vi "Add Parameter Channels with Definitions.vi"(6 "direction":T4, 8 "error in":errorcluster, 10 "parameters":T3(array[cluster]), 11 "message in":T1 format="%.0x") -> (0 "error out":errorcluster, 3 "message out":T1 format="%.0x")   [LabVIEW 2020, in "Ballard MIL-STD-1553 Scripting.lvlib"]
uses:
  Ballard MIL-STD-1553 Scripting.lvlib
  Shared/Direction.ctl
  <vilib>/NI VeriStand/Custom Device API/Custom Device Item Ref.ctl
  Shared/Parameter Definition.ctl
  <vilib>/NI VeriStand/Custom Device API/Custom Device Channel Type.ctl
  <vilib>/NI VeriStand/Custom Device API/Custom Device Channel.ctl
  <vilib>/NI VeriStand/Custom Device API/Custom Device API.lvlib
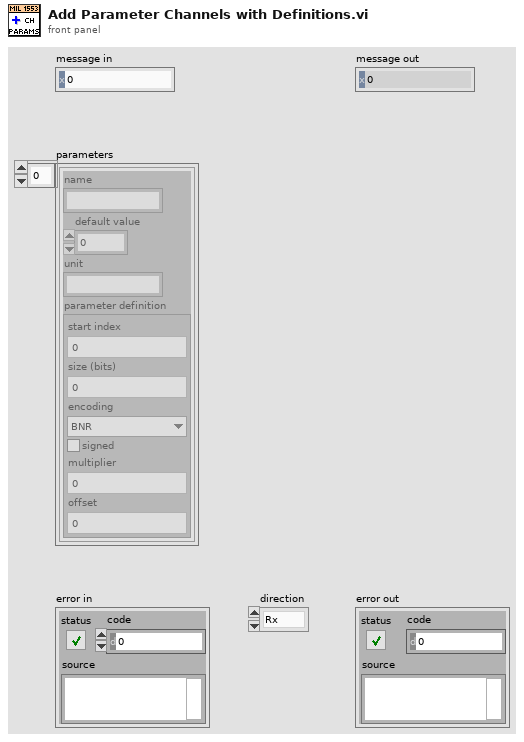
[diagram p1: front panel]
types:
  T1 = typedef "Custom Device API.lvlib/Custom Device Item Ref.ctl" = u64
  T2 = typedef "Parameter Definition.ctl" = cluster{"start index":i32, "size (bits)":i32, "encoding":enum16{"BNR", "BCD", "Discrete"}, "signed":bool, "multiplier":dbl, "offset":dbl}
  T3 = cluster{"name":string, "default value":dbl, "unit":string, "parameter definition":T2}[]
  T4 = typedef "Direction.ctl" = enum16{"Rx", "Tx"}
  T5 = typedef "Custom Device API.lvlib/Custom Device Channel Type.ctl" = enum16{"Input", "Output"}
  T6 = typedef "Custom Device API.lvlib/Custom Device Channel.ctl" = cluster{"Type":T5, "Units":string, "Default Value":dbl, "Faultable":bool, "Scalable":bool}
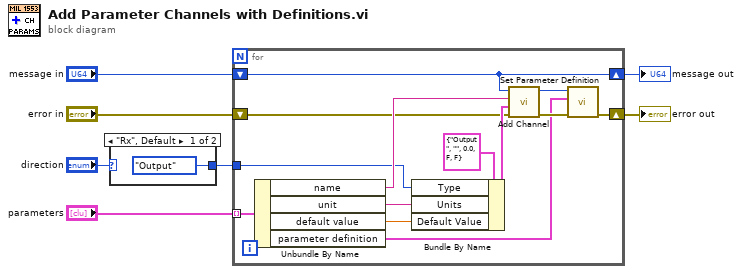
[diagram p0: block diagram]
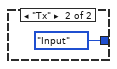
[diagram p2: hidden frame]
diagram:
  n1 = case shown="\"Rx\", Default" "direction" {
    tunnel: [Custom_Device_Channel_Type."Output" ("Type") Custom_Device_Channel_Type."Input" ("Type")] -> w1
    frame "Rx", Default {
    }
    frame "Tx" {
    }
  }
  n2 = for {
    shift-right: [w13] -> w7
    shift-left: "message in" -> [w13]
    tunnel: "parameters" -> [w22] mode=indexing
    shift-right: [w11] -> w6
    shift-left: "error in" -> [w12]
    tunnel: w1 -> [w10]
    n3 = Unbundle By Name(w22) -> ("name"=w18:string, "unit"=w20:string, "default value"=w19:dbl, "parameter definition"=w14:T2)
    n4 = Bundle By Name(cluster=T6 {"Type"=enum."Output", "Units"="", "Default Value"=0.0, "Faultable"=FALSE, "Scalable"=FALSE} ("Channel"), "Type"=w10, "Units"=w20, "Default Value"=w19) -> (w17:T6)
    n5 = call "Add Channel.vi"("error in"=w12, "Channel"=w17, "Name"=w18, "Frame Ref"=w13) -> ("error out"=w15:errorcluster, "Channel Ref out"=w16:T1)  [unwired: 6 in]
    n6 = call "Set Parameter Definition.vi"("error in"=w15, "parameter definition"=w14, "parameter in"=w16) -> ("error out"=w11:errorcluster)  [unwired: 7 in, 1 out]
  }
  "message out" <- w7
  "error out" <- w6
